vi "Build ID Strings.vi"(11 "Data Value ID":string) -> (2 "Type ID":string, 3 "Value ID":string)   [LabVIEW 2018, in "Test.lvclass"]
uses:
  Test.lvclass
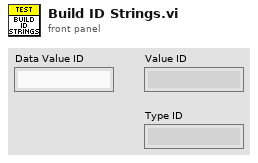
[diagram p1: front panel]
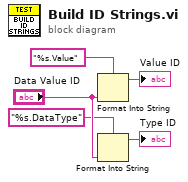
[diagram p0: block diagram]
diagram:
  n1 = Format Into String(format string="%s.Value", "Data Value ID") -> (resulting string=→"Value ID":string)  [unwired: 2 in, 1 out]
  n2 = Format Into String(format string="%s.DataType", "Data Value ID") -> (resulting string=→"Type ID":string)  [unwired: 2 in, 1 out]
